vi "Set Transfer Settings.vi"(8 "error in (no error)":errorcluster, 10 "settings":T1, 11 "transfer in":T3={"core"={"name"="Transfer"}, "component settings"=[], "channels"=[]} {"channels"."core"."string offset" format="%d bytes"}) -> (0 "error out":errorcluster, 3 "transfer out":T3={"core"={"name"="Transfer"}, "component settings"=[], "channels"=[]} {"channels"."core"."string offset" format="%d bytes"})   [LabVIEW 2017, in "DSF Core.lvlib" / "Configuration Session.lvclass"]
uses:
  Configuration Session.lvclass
  Typedefs/DSF Settings Info.ctl
  DSF Core.lvlib
  Typedefs/DSF Data Type.ctl
  Typedefs/DSF Engine Channel Configuration.ctl
  Typedefs/DSF Engine Transfer Configuration.ctl
  Typedefs/DSF Version Info.ctl
  Typedefs/DSF Core Channel Configuration.ctl
  Typedefs/DSF Core Transfer Configuration.ctl
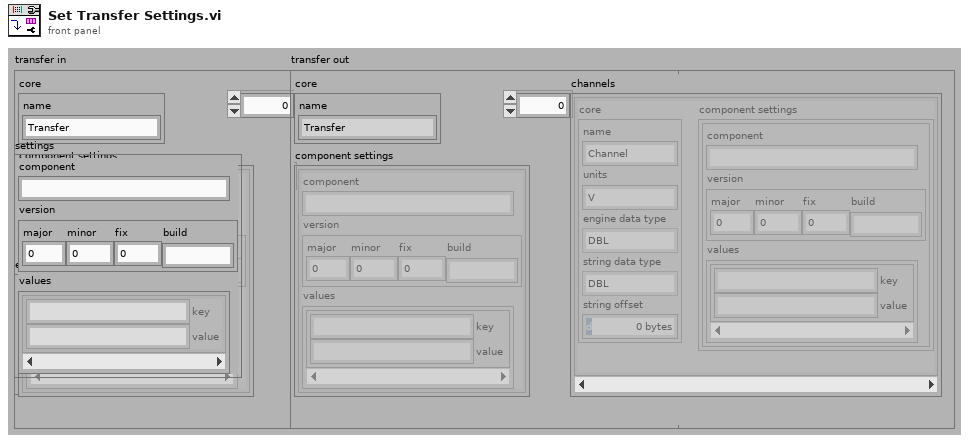
[diagram p1: front panel]
types:
  T1 = typedef "DSF Core.lvlib/DSF Settings Info.ctl" = cluster{"component":string, "version":T2, "values":cluster{"key":string, "value":string}[]}
  T2 = typedef "DSF Core.lvlib/DSF Version Info.ctl" = cluster{"major":u32, "minor":u32, "fix":u32, "build":string}
  T3 = typedef "DSF Core.lvlib/DSF Engine Transfer Configuration.ctl" = cluster{"core":T4, "component settings":T1[], "channels":T5[]}
  T4 = typedef "DSF Core.lvlib/DSF Core Transfer Configuration.ctl" = cluster{"name":string}
  T5 = typedef "DSF Core.lvlib/DSF Engine Channel Configuration.ctl" = cluster{"core":T6, "component settings":T1[]}
  T6 = typedef "DSF Core.lvlib/DSF Core Channel Configuration.ctl" = cluster{"name":string, "units":string, "engine data type":T7, "string data type":T7, "string offset":u64}
  T7 = typedef "DSF Core.lvlib/DSF Data Type.ctl" = enum8{"Bool", "SGL", "DBL", "I8", "I16", "I32", "I64", "U8", "U16", "U32", "U64"}
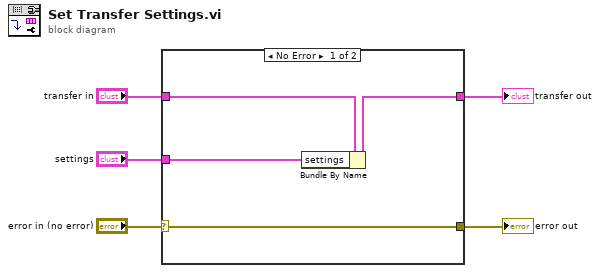
[diagram p0: block diagram]
diagram:
  n1 = case shown="No Error" "error in (no error)" {
    selector: "error in (no error)" -> [w7 w11]
    tunnel: [w7 w11] -> w5
    tunnel: [w8 w10] -> w3
    tunnel: "transfer in" -> [w9 w10]
    tunnel: "settings" -> [w6 _]
    frame No Error {
      n2 = Bundle By Name(cluster=w9, "settings"=w6) -> (w8:T3)
    }
    frame Error {
    }
  }
  "error out" <- w5
  "transfer out" <- w3
